vi "RequestOverride.vi"(8 "Error in":errorcluster[](array[cluster]), 11 "Visualize":refnum<class "VisualizeBase_class.lvclass">) -> (0 "Error out":errorcluster[](array[cluster]), 3 "RequestEvents":T1)   [LabVIEW 2014, in "Visualization.lvlib" / "VisualizeBase_class.lvclass"]
uses:
  VisualizeBase_class.lvclass
  clRequestEvents.ctl
  clUserEventType.ctl
  <userlib>/NIST/NISTErrorLib/NISTErrorLib.lvlib
panel:
  # "This dynamic terminal makes the vi overridable and is marked in the base class as \"Must Override\".  \n\nSo any child class derived from this parent class must override this VI"
  # "If you want to add other Request Events, open this typedef, copy an existing event and rename it to your event name."
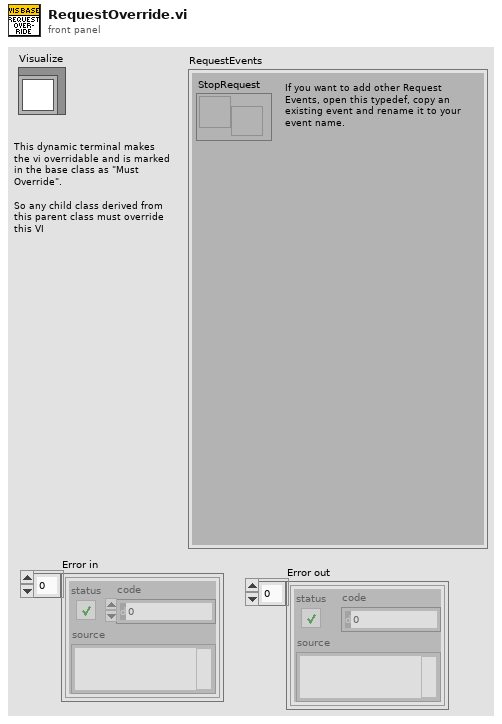
[diagram p1: front panel]
types:
  T1 = typedef "Visualization.lvlib/VisualizeBase_class.lvclass/clRequestEvents.ctl" = cluster{"StopRequest":refnum<user-event>}
  T2 = typedef "Visualization.lvlib/clRequestEvents.ctl" = cluster{"StopRequest":refnum<user-event>}
  T3 = typedef "Visualization.lvlib/VisualizeBase_class.lvclass/clUserEventType.ctl" = cluster{"BusIndex":i8, "Data":variant}
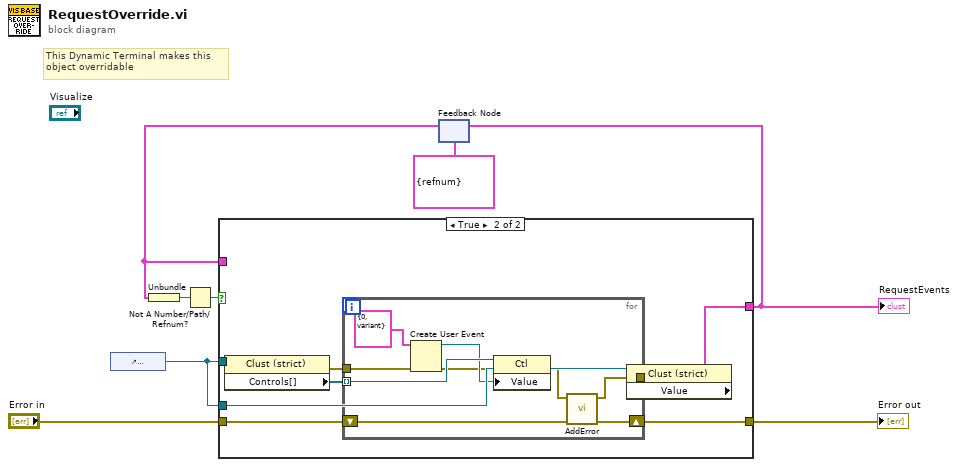
[diagram p0: block diagram]
diagram:
  # "This Dynamic Terminal makes this\nobject overridable"
  n1 = control-ref of="RequestEvents"() -> (w1:refnum<vi>)
  n2 = feedback #1(T1 {"StopRequest"=refnum} ("Value")) -> (w6:T2)
  n3 = Unbundle(w6) -> ("StopRequest"=w8:refnum<user-event>)
  n4 = Not A Number/Path/Refnum?(number/path/refnum=w8) -> (NaN/Path/Refnum?=w7:bool)
  n5 = case shown="True" w7 {
    tunnel: [w10 w13] -> w2
    tunnel: w6 -> [w10 _]
    tunnel: [w9 w15] -> w4
    tunnel: "Error in" -> [w9 w16]
    tunnel: w1 -> [_ w12]
    tunnel: w1 -> [_ w11]
    frame False {
    }
    frame True {
      n6 = property on="Property Node" class="Clust (strict)"(reference=w12) -> (error out=w17:errorcluster, "Controls[]"=w18:refnum<vi>[])  [unwired: 1 in, 1 out]
      n7 = for {
        tunnel: w18 -> [w25] mode=indexing
        tunnel: w17 -> [w26]
        shift-right: [w20] -> w15
        shift-left: w16 -> [w21]
        tunnel: [w19] -> w14
        n8 = Create User Event(user event datatype=T3 {"BusIndex"=0, "Data"=variant} ("clEventType"), error in=w26) -> (user event=w24:refnum<user-event>, error out=w23:errorcluster)
        n9 = property class="Ctl"(reference=w25, error in=w23, "Value"=w24) -> (error out=w22:errorcluster)  [unwired: 1 out]
        n10 = call <userlib>:"AddError.vi"("ErrorArray"=w21, "error in (no error)"=w22) -> ("ErrorArray"=w20:errorcluster[], "error out"=w19:errorcluster)  [unwired: 8 in]
      }
      n11 = property on="Property Node" class="Clust (strict)"(reference=w11, error in=w14) -> ("Value"=w13:T2)  [unwired: 2 out]
    }
  }
  "Error out" <- w4
  "RequestEvents" <- w2
  n12 = feedback-in #1(w2) -> ()
